vi "Initialise Slylandro.vi"(8 "error in (no error)":errorcluster, 11 "Renderer":u32) -> (0 "error out":errorcluster, 3 "Ship out":refnum<class "Slylandro.lvclass">)   [LabVIEW 2021, in "Slylandro.lvclass"]
uses:
  Slylandro.lvclass
  Ship/Config.ctl
  Ship/Ship.lvclass
  Element/Element.lvclass
  Motion/Motion.lvclass
  Vector 2D/Vector 2D.lvclass
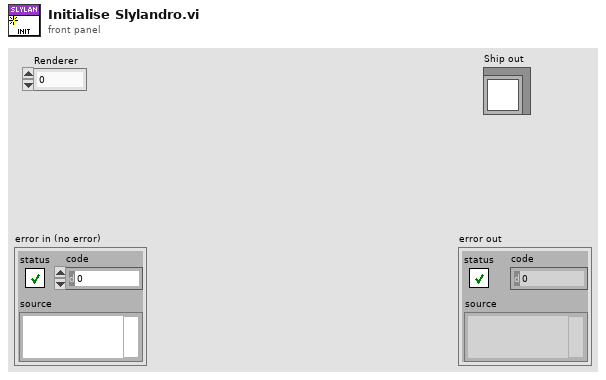
[diagram p1: front panel]
types:
  T1 = typedef "Ship.lvclass/Config.ctl" = cluster{"Race":string, "Ship Name":string, "Max Crew":i32, "Max Energy":i32, "Energy Regeneration":i32, "Weapon Energy Cost":i32, "Special Energy Cost":i32, "Energy Wait":i32, "Max Thrust":i32, "Thrust Increment":i32, "Turn Wait":i32, "Thrust Wait":i32, "Weapon Wait":i32, "Special Wait":i32, "Ship Mass":i32}
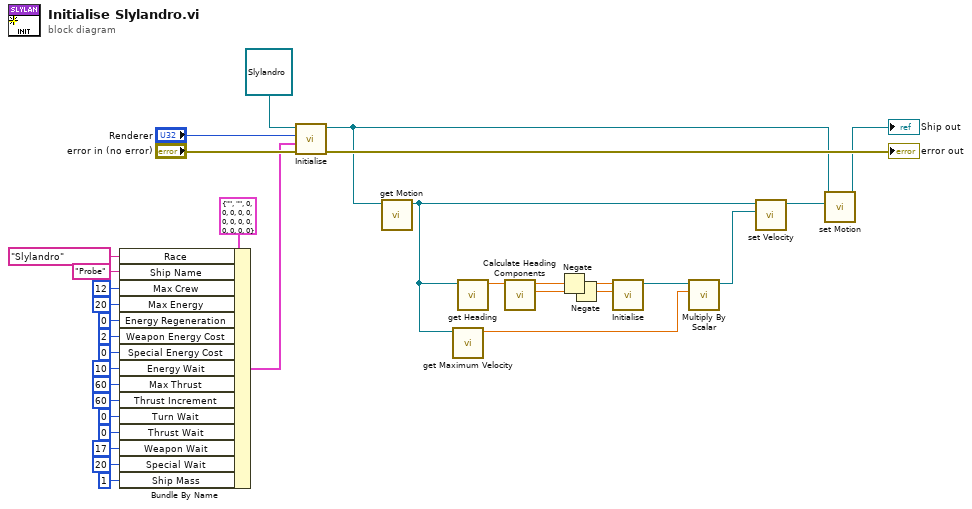
[diagram p0: block diagram]
diagram:
  n1 = Bundle By Name(cluster=T1 {"Race"="", "Ship Name"="", "Max Crew"=0, "Max Energy"=0, "Energy Regeneration"=0, "Weapon Energy Cost"=0, "Special Energy Cost"=0, "Energy Wait"=0, "Max Thrust"=0, "Thrust Increment"=0, "Turn Wait"=0, "Thrust Wait"=0, "Weapon Wait"=0, "Special Wait"=0, "Ship Mass"=0} ("Common"), "Race"="Slylandro" ("name or relative path"), "Ship Name"="Probe", "Max Crew"=12, "Max Energy"=20, "Energy Regeneration"=0, "Weapon Energy Cost"=2, "Special Energy Cost"=0, "Energy Wait"=10, "Max Thrust"=60, "Thrust Increment"=60, "Turn Wait"=0, "Thrust Wait"=0, "Weapon Wait"=17, "Special Wait"=20, "Ship Mass"=1) -> (w31:T1)
  n2 = call-dynamic "Initialise.vi"("error in (no error)"="error in (no error)", "Common"=w31, "Renderer"="Renderer", "Ship in"=refnum<class "Slylandro.lvclass"> refnum ("Ship")) -> ("error out"=→"error out":errorcluster, "Ship out"=w4:refnum<class "Slylandro.lvclass">)  [unwired: 6 in]
  n3 = call "get Motion.vi"("Element in"=w4) -> ("Motion"=w2:refnum<class "Motion.lvclass">)  [unwired: 10 in]
  n4 = call "get Maximum Velocity.vi"("Motion in"=w2) -> ("Maximum Velocity"=w1:sgl)  [unwired: 10 in]
  n5 = call "get Heading.vi"("Motion in"=w2) -> ("Heading [deg]"=w6:sgl)  [unwired: 10 in]
  n6 = call "Calculate Heading Components.vi"("Heading In [deg]"=w6) -> ("Sin Heading"=w9:sgl, "Cos Heading"=w8:sgl)  [unwired: 9 in]
  n7 = Negate(x=w8) -> (-x=w11:sgl)
  n8 = Negate(x=w9) -> (-x=w12:sgl)
  n9 = call "Initialise.vi"("y"=w12, "x"=w11) -> ("Vector 2D out"=w10:refnum<class "Vector 2D.lvclass">)  [unwired: 9 in]
  n10 = call "Multiply By Scalar.vi"("x"=w1, "A"=w10) -> ("Ax"=w7:refnum<class "Vector 2D.lvclass">)  [unwired: 9 in]
  n11 = call "set Velocity.vi"("Velocity"=w7, "Motion in"=w2) -> ("Motion out"=w5:refnum<class "Motion.lvclass">)  [unwired: 9 in]
  n12 = call "set Motion.vi"("Motion"=w5, "Element in"=w4) -> ("Element out"=→"Ship out":refnum<class "Slylandro.lvclass">)  [unwired: 9 in]
